vi "Dashboard Loop.vi"() -> ()   [LabVIEW 2013]
uses:
  Common Code/Dashboard UDP/Indicator Packet.ctl
  Common Code/Dashboard UDP/Auton Indicators.ctl
  Common Code/Dashboard UDP/Roller Indicators.ctl
  Common Code/IR Logic State.ctl
  Common Code/Dashboard UDP/Shooter Indicators.ctl
  Common Code/Shooter State.ctl
  Common Code/Dashboard UDP/Halo Indicators.ctl
  Common Code/Dashboard UDP/Drive Indicators.ctl
  Sensors/Encoder Data.ctl
  Sensors/Single Encoder Data.ctl
  Common Code/Vision Mode.ctl
  Drivetrain/DT Mode.ctl
  Rollers/Roller Mode.ctl
  Robot Global Data.vi
  <vilib>/Rock Robotics/WPI/Gyro/WPI_GyroRefNum Registry Get.vi
  <vilib>/Rock Robotics/WPI/Gyro/WPI_GyroGetAngle.vi
  <vilib>/Rock Robotics/WPI/DigitalInput/WPI_DigitalInputRefNum Registry Get.vi
  <vilib>/Rock Robotics/WPI/DigitalInput/WPI_DigitalInputGetValue.vi
panel:
  out "Indicator Packet":T1={"Gyro/Steer Target"=0.0, "Gyro/In Range"=FALSE, "Gyro Heading"=0.0, "Auton/Files"="", "Auton Indicators"={"DistDrive/Steer"=FALSE, "DistDrive/Y Check"=FALSE, "Auton/Left Hot"=FALSE, "Auton/Right Hot"=FALSE, "DistDrive/Y Dist"=0.0, "DistDrive/Y Target"=0.0, "DistDrive/X Dist"=0.0, "DistDrive/X Target"=0.0, "Gyro Heading"=0.0, "DistDrive/Steer Target"=0.0, "DistDrive/X Check"=FALSE, "Auton/Hot Found"=FALSE, "Auton/Goals Used"=0.0, "Auton/Total Commands"=0.0, "Auton/Current Command"=0.0, "Auton/File"=0.0}, "Heartbeat"=0.0, "100ms Loop Time"=0, "IR Dist/Line Detected Left"=FALSE, "IR Dist/Line Detected Right"=FALSE, "Roller Indicators"={"Roller/Front IR"=FALSE, "Roller/Center IR"=FALSE, "Roller/Back IR"=FALSE, "Roller/IR State"=enum."Waiting", "Roller/Auto Enabled"=FALSE, "Roller/Hold"=FALSE, "Roller/Net Solenoid"=FALSE}, "Shooter/Indicators"={"Pressure/Line"=-1.0, "Pressure/Shooter"=-1.0, "Shooter/Release"=FALSE, "Shooter/Trigger"=FALSE, "Shooter/Retracted"=FALSE, "Shooter/Ready"=FALSE, "Shooter/Add"=FALSE, "Shooter/State"=enum."Wait", "Shooter/Punch"=FALSE, "Shooter/High"=FALSE, "Shooter/AutoPunch"=FALSE}, "Halo/Indicators"={"Halo"=FALSE, "Roller Halo"=FALSE, "Shooter Halo"=FALSE, "Auto Halo"=FALSE, "Manual Halo"=FALSE}, "Drive Indicators"={"Drive/Throttle"=0.0, "Drive/Steer"=0.0, "Drive/Translation X"=0.0, "Drive/Omni"=FALSE, "Roller/Front Output"=0.0, "Roller/Back Output"=0.0, "Roller/Front Solenoid"=FALSE, "Roller/Back Solenoid"=FALSE, "Drive/Gear"=0.0}, "Encoder Data"={"Avg Distance L/R"=0.0, "Avg Speed L/R"=0.0, "Left"={"Distance"=0.0, "Speed"=0.0, "Ticks"=0.0}, "Right"={"Distance"=0.0, "Speed"=0.0, "Ticks"=0.0}, "Omni"={"Distance"=0.0, "Speed"=0.0, "Ticks"=0.0}}, "Vision Mode "=enum."Normal", "Drivetrain Mode"=enum."Manual"} {"Encoder Data"."Omni"."Ticks" format="%#.6g"; "Encoder Data"."Right"."Ticks" format="%#.6g"; "Encoder Data"."Left"."Ticks" format="%#.6g"; "Drive Indicators"."Roller/Back Output" scale=-1.0..1.0; "Drive Indicators"."Roller/Front Output" scale=-1.0..1.0; "Drive Indicators"."Drive/Translation X" scale=-1.0..1.0; "Drive Indicators"."Drive/Steer" scale=-1.0..1.0; "Drive Indicators"."Drive/Throttle" scale=-1.0..1.0}
  # "IR"
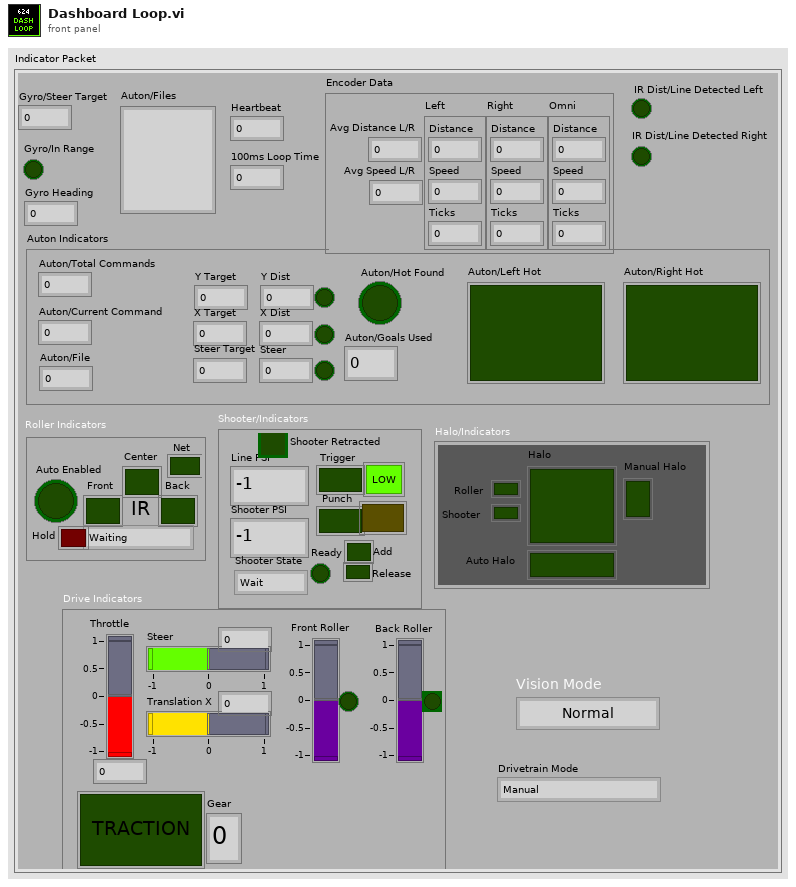
[diagram p1: front panel]
types:
  T1 = typedef "Indicator Packet.ctl" = cluster{"Gyro/Steer Target":dbl, "Gyro/In Range":bool, "Gyro Heading":dbl, "Auton/Files":string, "Auton Indicators":T2, "Heartbeat":dbl, "100ms Loop Time":i32, "IR Dist/Line Detected Left":bool, "IR Dist/Line Detected Right":bool, "Roller Indicators":T3, "Shooter/Indicators":T5, "Halo/Indicators":T7, "Drive Indicators":T8, "Encoder Data":T9, "Vision Mode ":T11, "Drivetrain Mode":T12}
  T2 = typedef "Auton Indicators.ctl" = cluster{"DistDrive/Steer":bool, "DistDrive/Y Check":bool, "Auton/Left Hot":bool, "Auton/Right Hot":bool, "DistDrive/Y Dist":dbl, "DistDrive/Y Target":dbl, "DistDrive/X Dist":dbl, "DistDrive/X Target":dbl, "Gyro Heading":dbl, "DistDrive/Steer Target":dbl, "DistDrive/X Check":bool, "Auton/Hot Found":bool, "Auton/Goals Used":dbl, "Auton/Total Commands":dbl, "Auton/Current Command":dbl, "Auton/File":dbl}
  T3 = typedef "Roller Indicators.ctl" = cluster{"Roller/Front IR":bool, "Roller/Center IR":bool, "Roller/Back IR":bool, "Roller/IR State":T4, "Roller/Auto Enabled":bool, "Roller/Hold":bool, "Roller/Net Solenoid":bool}
  T4 = typedef "IR Logic State.ctl" = enum16{"Waiting", "Requested", "Loading", "Full", "Wait for Center", "Carry", "Full Carry", "Holding"}
  T5 = typedef "Shooter Indicators.ctl" = cluster{"Pressure/Line":dbl, "Pressure/Shooter":dbl, "Shooter/Release":bool, "Shooter/Trigger":bool, "Shooter/Retracted":bool, "Shooter/Ready":bool, "Shooter/Add":bool, "Shooter/State":T6, "Shooter/Punch":bool, "Shooter/High":bool, "Shooter/AutoPunch":bool}
  T6 = typedef "Shooter State.ctl" = enum16{"Wait", "Fill Piston", "Lift Halo", "Trigger", "Reset", "Soft Release", "Soft Unpin", "Soft Refill", "Soft Shoot", "Toss Prep", "Toss Release"}
  T7 = typedef "Halo Indicators.ctl" = cluster{"Halo":bool, "Roller Halo":bool, "Shooter Halo":bool, "Auto Halo":bool, "Manual Halo":bool}
  T8 = typedef "Drive Indicators.ctl" = cluster{"Drive/Throttle":dbl, "Drive/Steer":dbl, "Drive/Translation X":dbl, "Drive/Omni":bool, "Roller/Front Output":dbl, "Roller/Back Output":dbl, "Roller/Front Solenoid":bool, "Roller/Back Solenoid":bool, "Drive/Gear":dbl}
  T9 = typedef "Encoder Data.ctl" = cluster{"Avg Distance L/R":dbl, "Avg Speed L/R":dbl, "Left":T10, "Right":T10, "Omni":T10}
  T10 = typedef "Single Encoder Data.ctl" = cluster{"Distance":dbl, "Speed":dbl, "Ticks":dbl}
  T11 = typedef "Vision Mode.ctl" = enum16{"Normal", "Extreme Left", "Extreme Right"}
  T12 = typedef "DT Mode.ctl" = enum16{"Manual", "Gyro Steer", "Distance Drive", "Fieldcentric", "Roll Maneuver", "Alt Roll Maneuver"}
  T13 = typedef "Roller Mode.ctl" = enum16{"None", "Front", "Back", "Both", "Manual"}
  T14 = typedef "WPI_DriverStationRobotMode2.ctl" = enum16{"Autonomous Disabled", "Autonomous Enabled", "Teleop Disabled", "Teleop Enabled", "Timeout", "Finish", "Test Disabled", "Test Enabled"}
  T15 = typedef "Roller Control.ctl" = cluster{"Mode":T13, "Front":enum16{"Stop", "Forward", "Reverse"}, "Back":enum16{"Stop", "Forward", "Reverse"}, "Reset":bool, "Front Piston":bool, "Halo":bool, "Net Piston":bool, "Carry Two":bool, "Hold":bool}
  T16 = typedef "Drivetrain Status.ctl" = cluster{"Mode":T12, "X":dbl, "Y":dbl, "Steer":dbl, "Low Gear":bool, "Omni":bool}
  T17 = typedef "Roller Status.ctl" = cluster{"State":T4, "Front Power":dbl, "Front Solenoid":bool}
  T18 = typedef "Distance Drive Result.ctl" = cluster{"Finished":bool, "distance target":cluster{"x":dbl, "y":dbl}, "Heading Target":dbl, "X Check":bool, "Y Check":bool, "X Dist":dbl, "Y Dist":dbl}
  T19 = typedef "Shooter Manual Control.ctl" = cluster{"Command":T20, "Offset":dbl, "Trigger":bool, "Add":bool, "Release":bool, "Reset":bool, "Target Pressure":dbl, "Punch":bool, "AutoPunch":bool}
  T20 = typedef "Shooter Command.ctl" = enum16{"None", "Warmup", "Shoot", "Line Shoot", "Soft Shoot", "Toss"}
  T21 = typedef "Dashboard UDP Packet.ctl" = cluster{"Camera":T22, "Gyro":T23, "Encoder":T25, "Auto Shift":T26, "Auton":T27, "Drive/Ramp X":dbl, "Drive/Ramp Y":dbl, "Drive/Battery Cutoff":dbl, "Pressure/Compressor Min Voltage":dbl, "Pressure/Compressor Delay":dbl, "Controller/Strafe Correction":bool, "Shooter":T28, "Rollers":T29, "Abort":bool, "Finish":bool, "IR Halo Sustain Time":dbl, "Disable Compressor":bool, "Center Omni Drive Delay":i32, "Vision Mode":T11, "Radius Throttle":bool, "Fieldcentric":T30, "Roll":T31, "Stick Deadband":dbl}
  T22 = typedef "Camera Controls.ctl" = cluster{"Camera/View Angle X":dbl, "Camera/Goal Track Timeout":dbl, "Camera/View Angle Y":dbl, "Camera/Goal Exposure":dbl, "Camera/Vision Receive Timeout":dbl, "Camera/Offset 1":dbl, "Camera/Offset 2":dbl}
  T23 = typedef "Gyro Controls.ctl" = cluster{"Gyro/Angle Tolerance":dbl, "Gyro/Steer Closeness Threshold":dbl, "Steer PID":T24, "Steer Close PID":T24}
  T24 = typedef "PID Params.ctl" = cluster{"max":dbl, "min":dbl, "P":dbl, "I":dbl, "D":dbl}
  T25 = typedef "Encoder Controls.ctl" = cluster{"Encoders/Reset":bool, "Encoders/Omni Constant":dbl, "Encoders/Omni Tick Constant":dbl, "Encoders/Left Constant":dbl, "Encoders/Right Constant":dbl, "Encoders/Right Tick Constant":dbl}
  T26 = typedef "Auto Shift Controls.ctl" = cluster{"AutoShift/Upshift Throttle Accel":dbl, "AutoShift/Speed Threshold":dbl, "AutoShift/Upshift Throttle":dbl, "AutoShift/Upshift Accel":dbl, "AutoShift/Downshift Accel":dbl, "AutoShift/Downshift Throttle":dbl, "AutoShift/Delay":dbl, "AutoShift/Enabled":bool}
  T27 = typedef "Auton Controls.ctl" = cluster{"Auton/Left Shoot X-Coord":dbl, "Auton/Right Shoot X-Coord":dbl, "DistDrive/Distance Stop Threshold":dbl, "DistDrive/Max Stop Speed":dbl, "Auton/Back Piston Time":dbl, "Auton/Manual Hot":bool, "Auton/Manual Hot Right":bool, "Default X PID":T24, "Default Y PID":T24, "Half Over Delay":dbl}
  T28 = typedef "Shooter Controls.ctl" = cluster{"Shooter/Reset Time":dbl, "Shooter/Release Delay":dbl, "Shooter/Pressure Steady Time":dbl, "Shooter/Misfire Delay":dbl, "Shooter/Ball Settle Time":dbl, "Shooter/Line IR Delay":dbl, "Pressure/Upper PSI Time":dbl, "Pressure/Lower PSI Time":dbl, "Shooter/Punch Delay":dbl, "Shooter/Target Pressure":dbl, "Pressure/Line B":dbl, "Pressure/Line M":dbl, "Pressure/Shooter M":dbl, "Pressure/Shooter B":dbl, "Halo Time":dbl, "Soft Release Delay":dbl, "Soft Unpin Delay":dbl, "Soft Shoot Delay":dbl, "Toss Release Time":dbl}
  T29 = typedef "Roller Controls.ctl" = cluster{"Roller/Load IRs Verify Time":dbl, "Roller/Center IR Latch Time":dbl, "Roller/Speed Front":dbl, "Roller/Speed Back":dbl, "Roller/Entry Timeout":dbl, "Roller/To Center Timeout":dbl, "Roller/Sustain Time":dbl, "Roller/Verify Center Time":dbl}
  T30 = typedef "Fieldcentric Controls.ctl" = cluster{"Relative Angle":bool, "Point Robot":bool, "X/Y ratio low":dbl, "Steering Gain":dbl, "Force Omni Down":bool, "Enable":bool, "X/Y ratio high":dbl}
  T31 = typedef "Roll Maneuver.ctl" = cluster{"X 1":dbl, "Y 1":dbl, "Y 2":dbl, "X 2":dbl, "Y 3":dbl, "X 3":dbl, "Time 1":i32, "Time 2":i32, "Time 3":i32, "Angle Start":dbl, "Angle End":dbl, "Angle Linearity":dbl}
  T32 = typedef "Shooter Status.ctl" = cluster{"Shooter Ready":bool, "Add":bool, "Punch":bool, "Release":bool, "Trigger":bool, "High":bool, "State":T6}
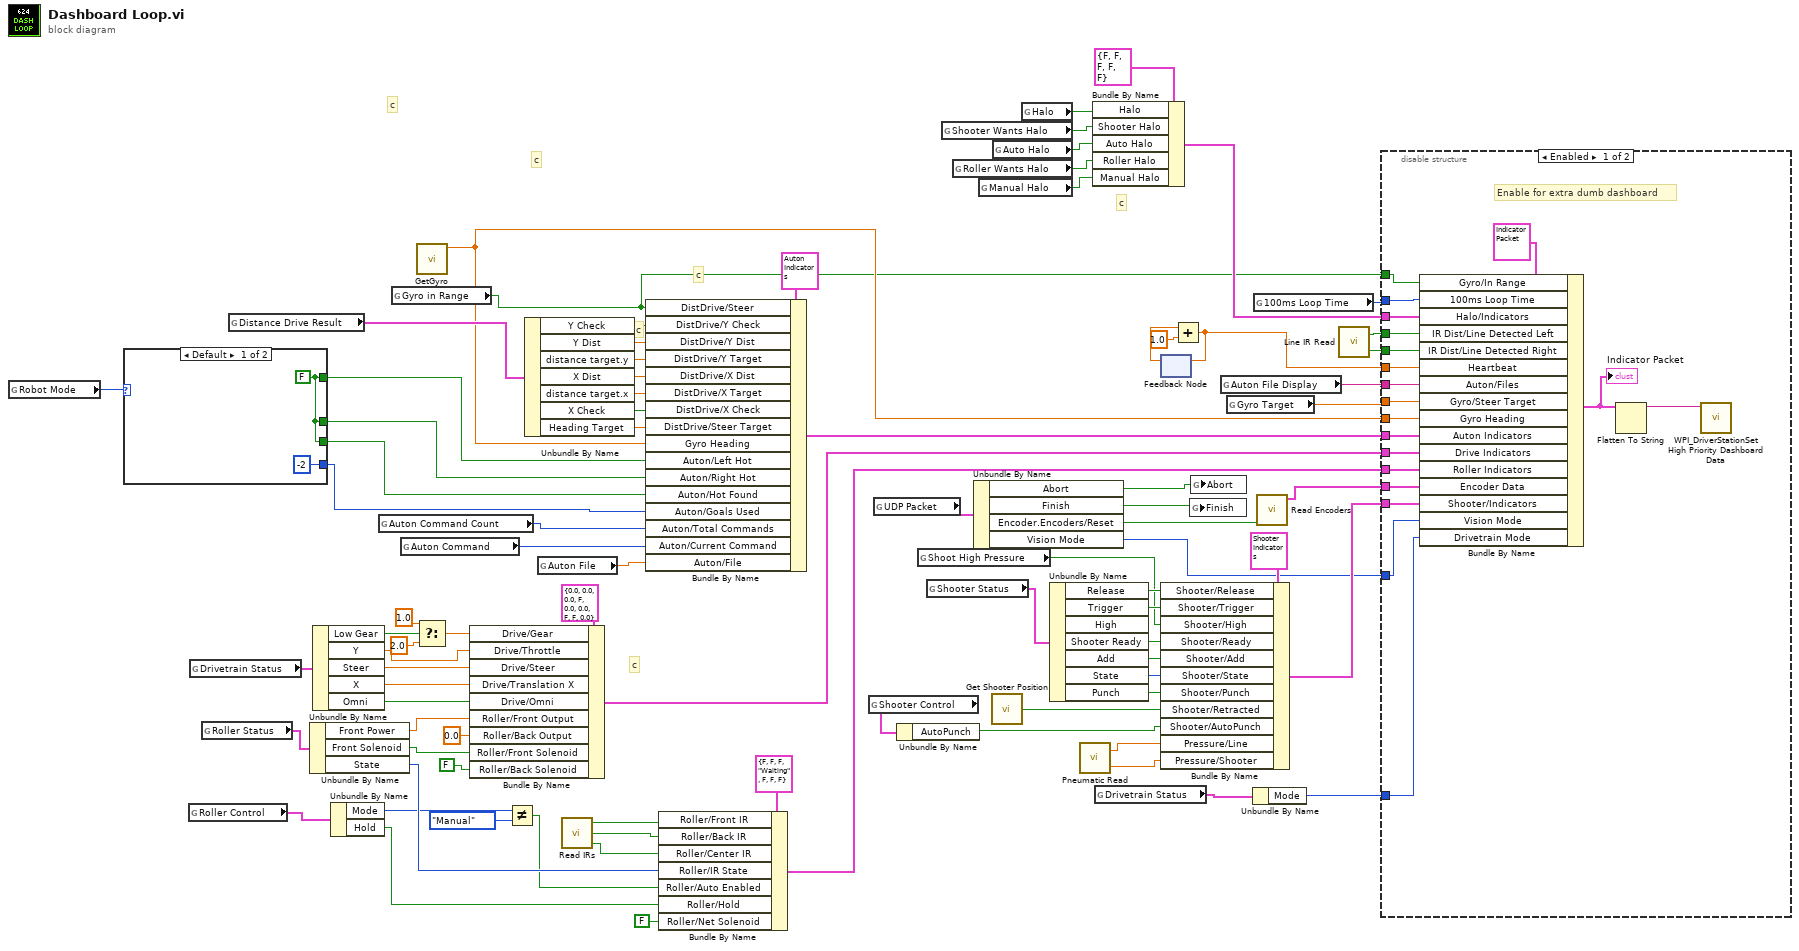
[diagram p0: block diagram]
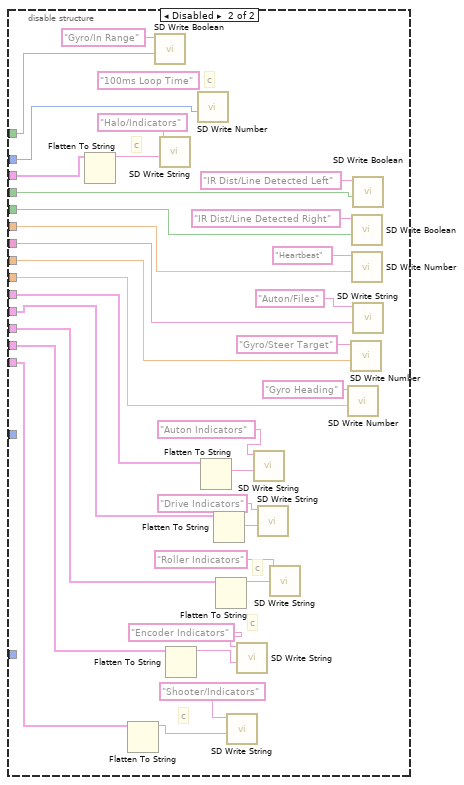
[diagram p2: hidden frame]
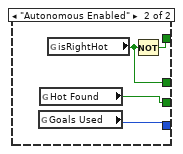
[diagram p3: hidden frame]
diagram:
  # "c"
  # "c"
  # "c"
  # "c"
  # "c"
  # "c"
  n1 = global read "Robot Global Data.vi" "Robot Mode"() -> (w82:T14)
  n2 = case shown="Default" w82 {
    tunnel: [w88 w92] -> w33
    tunnel: [w88 w91] -> w34
    tunnel: [w88 w90] -> w35
    tunnel: [-2 ("Goals Used") w89] -> w36
    frame Default {
      w88 = FALSE
    }
    frame "Autonomous Enabled" {
      n3 = global read "Robot Global Data.vi" "Goals Used"() -> (w89:i32)
      n4 = global read "Robot Global Data.vi" "Hot Found"() -> (w90:bool)
      n5 = global read "Robot Global Data.vi" "isRightHot"() -> (w91:bool)
      n6 = Not(x=w91) -> (.not. x?=w92:bool)
    }
  }
  n7 = global read "Robot Global Data.vi" "Roller Control"() -> (w57:T15)
  n8 = global read "Robot Global Data.vi" "Drivetrain Status"() -> (w76:T16)
  n9 = global read "Robot Global Data.vi" "Roller Status"() -> (w69:T17)
  n10 = global read "Robot Global Data.vi" "Distance Drive Result"() -> (w32:T18)
  n11 = Unbundle By Name(w69) -> ("Front Power"=w67:dbl, "Front Solenoid"=w68:bool, "State"=w61:T4)
  n12 = Unbundle By Name(w76) -> ("Low Gear"=w75:bool, "Y"=w73:dbl, "Steer"=w72:dbl, "X"=w71:dbl, "Omni"=w70:bool)
  n13 = Unbundle By Name(w57) -> ("Mode"=w56:T13, "Hold"=w53:bool)
  n14 = global read "Robot Global Data.vi" "Auton Command Count"() -> (w37:i32)
  n15 = global read "Robot Global Data.vi" "Gyro in Range"() -> (w5:bool)
  n16 = global read "Robot Global Data.vi" "Auton Command"() -> (w38:i32)
  n17 = call "GetGyro.vi"() -> ("Angle"=w13:dbl)  [unwired: 9 in, 2 out]
  n18 = Select(t=1.0, s=w75, f=2.0) -> (s? t:f=w74:dbl)
  n19 = Bundle By Name(cluster=T8 {"Drive/Throttle"=0.0, "Drive/Steer"=0.0, "Drive/Translation X"=0.0, "Drive/Omni"=FALSE, "Roller/Front Output"=0.0, "Roller/Back Output"=0.0, "Roller/Front Solenoid"=FALSE, "Roller/Back Solenoid"=FALSE, "Drive/Gear"=0.0} ("Drive Indicators"), "Drive/Gear"=w74, "Drive/Throttle"=w73, "Drive/Steer"=w72, "Drive/Translation X"=w71, "Drive/Omni"=w70, "Roller/Front Output"=w67, "Roller/Back Output"=0.0, "Roller/Front Solenoid"=w68, "Roller/Back Solenoid"=FALSE) -> (w11:T8)
  n20 = Not Equal?(x=w56, y=Roller_Mode."Manual") -> (x != y?=w54:bool)
  n21 = Unbundle By Name(w32) -> ("Y Check"=w25:bool, "Y Dist"=w26:dbl, "distance target.y"=w27:dbl, "X Dist"=w28:dbl, "distance target.x"=w29:dbl, "X Check"=w30:bool, "Heading Target"=w31:dbl)
  n22 = global read "Robot Global Data.vi" "Auton File"() -> (w39:dbl)
  n23 = call "Read IRs.vi"() -> ("Center"=w58:bool, "Back"=w59:bool, "Front"=w60:bool)  [unwired: 2 in, 1 out]
  n24 = Bundle By Name(cluster=T2 {"DistDrive/Steer"=FALSE, "DistDrive/Y Check"=FALSE, "Auton/Left Hot"=FALSE, "Auton/Right Hot"=FALSE, "DistDrive/Y Dist"=0.0, "DistDrive/Y Target"=0.0, "DistDrive/X Dist"=0.0, "DistDrive/X Target"=0.0, "Gyro Heading"=0.0, "DistDrive/Steer Target"=0.0, "DistDrive/X Check"=FALSE, "Auton/Hot Found"=FALSE, "Auton/Goals Used"=0.0, "Auton/Total Commands"=0.0, "Auton/Current Command"=0.0, "Auton/File"=0.0} ("Auton Indicators"), "DistDrive/Steer"=w5, "DistDrive/Y Check"=w25, "DistDrive/Y Dist"=w26, "DistDrive/Y Target"=w27, "DistDrive/X Dist"=w28, "DistDrive/X Target"=w29, "DistDrive/X Check"=w30, "DistDrive/Steer Target"=w31, "Gyro Heading"=w13, "Auton/Left Hot"=w33, "Auton/Right Hot"=w34, "Auton/Hot Found"=w35, "Auton/Goals Used"=w36, "Auton/Total Commands"=w37, "Auton/Current Command"=w38, "Auton/File"=w39) -> (w12:T2)
  n25 = Bundle By Name(cluster=T3 {"Roller/Front IR"=FALSE, "Roller/Center IR"=FALSE, "Roller/Back IR"=FALSE, "Roller/IR State"=enum."Waiting", "Roller/Auto Enabled"=FALSE, "Roller/Hold"=FALSE, "Roller/Net Solenoid"=FALSE} ("Roller Indicators"), "Roller/Front IR"=w60, "Roller/Back IR"=w59, "Roller/Center IR"=w58, "Roller/IR State"=w61, "Roller/Auto Enabled"=w54, "Roller/Hold"=w53, "Roller/Net Solenoid"=FALSE) -> (w10:T3)
  n26 = global read "Robot Global Data.vi" "Shooter Control"() -> (w81:T19)
  n27 = global read "Robot Global Data.vi" "UDP Packet"() -> (w80:T21)
  n28 = Unbundle By Name(w81) -> ("AutoPunch"=w43:bool)
  n29 = global read "Robot Global Data.vi" "Shoot High Pressure"() -> (w24:bool)
  n30 = global read "Robot Global Data.vi" "Shooter Status"() -> (w51:T32)
  n31 = global read "Robot Global Data.vi" "Shooter Wants Halo"() -> (w19:bool)
  n32 = global read "Robot Global Data.vi" "Roller Wants Halo"() -> (w21:bool)
  n33 = Unbundle By Name(w80) -> ("Abort"=w79:bool, "Finish"=w78:bool, "Encoder.Encoders/Reset"=w77:bool, "Vision Mode"=w3:T11)
  n34 = global read "Robot Global Data.vi" "Manual Halo"() -> (w22:bool)
  n35 = call "Get Shooter Position.vi"() -> ("Is Retracted"=w44:bool)  [unwired: 1 in]
  n36 = global read "Robot Global Data.vi" "Auto Halo"() -> (w20:bool)
  n37 = global read "Robot Global Data.vi" "Halo"() -> (w18:bool)
  n38 = Unbundle By Name(w51) -> ("Release"=w50:bool, "Trigger"=w49:bool, "Shooter Ready"=w48:bool, "Add"=w47:bool, "State"=w46:T6, "Punch"=w45:bool)  [unwired: 1 out]
  n39 = call "Pneumatic Read.vi"() -> ("Shooter"=w41:dbl, "Line"=w42:dbl)  [unwired: 2 in]
  n40 = Bundle By Name(cluster=T7 {"Halo"=FALSE, "Roller Halo"=FALSE, "Shooter Halo"=FALSE, "Auto Halo"=FALSE, "Manual Halo"=FALSE} ("Halo Indicators"), "Halo"=w18, "Shooter Halo"=w19, "Auto Halo"=w20, "Roller Halo"=w21, "Manual Halo"=w22) -> (w16:T7)
  n41 = global read "Robot Global Data.vi" "Drivetrain Status"() -> (w2:T16)
  n42 = feedback #1() -> (w85:dbl)  [unwired: 1 in]
  n43 = Bundle By Name(cluster=T5 {"Pressure/Line"=-1.0, "Pressure/Shooter"=-1.0, "Shooter/Release"=FALSE, "Shooter/Trigger"=FALSE, "Shooter/Retracted"=FALSE, "Shooter/Ready"=FALSE, "Shooter/Add"=FALSE, "Shooter/State"=enum."Wait", "Shooter/Punch"=FALSE, "Shooter/High"=FALSE, "Shooter/AutoPunch"=FALSE} ("Shooter Indicators"), "Shooter/Release"=w50, "Shooter/Trigger"=w49, "Shooter/High"=w24, "Shooter/Ready"=w48, "Shooter/Add"=w47, "Shooter/State"=w46, "Shooter/Punch"=w45, "Shooter/Retracted"=w44, "Shooter/AutoPunch"=w43, "Pressure/Line"=w42, "Pressure/Shooter"=w41) -> (w9:T5)
  n44 = Add(x=w85, y=1.0) -> (x+y=w15:dbl)
  n45 = feedback-in #1(w15) -> ()
  n46 = global write "Robot Global Data.vi" "Finish"(w78) -> ()
  n47 = global write "Robot Global Data.vi" "Abort"(w79) -> ()
  n48 = global read "Robot Global Data.vi" "Auton File Display"() -> (w6:string)
  n49 = global read "Robot Global Data.vi" "Gyro Target"() -> (w14:dbl)
  n50 = Unbundle By Name(w2) -> ("Mode"=w1:T12)
  n51 = global read "Robot Global Data.vi" "100ms Loop Time"() -> (w17:i32)
  n52 = call "Read Encoders.vi"("Reset"=w77) -> ("Encoder Data"=w4:T9)  [unwired: 10 in]
  n53 = call "Line IR Read.vi"() -> ("Line IR Right"=w7:bool, "Line IR Left"=w8:bool)  [unwired: 2 in]
  n54 = disable-structure shown="Enabled" {
    disable-tunnel: w17 -> [w110 w144]
    disable-tunnel: w16 -> [w109 w141]
    disable-tunnel: w8 -> [w108 w139]
    disable-tunnel: w7 -> [w107 w138]
    disable-tunnel: w15 -> [w106 w135]
    disable-tunnel: w6 -> [w105 w133]
    disable-tunnel: w14 -> [w104 w131]
    disable-tunnel: w13 -> [w103 w129]
    disable-tunnel: w12 -> [w102 w126]
    disable-tunnel: w11 -> [w101 w120]
    disable-tunnel: w10 -> [w100 w123]
    disable-tunnel: w4 -> [w95 w117]
    disable-tunnel: w9 -> [w99 w114]
    disable-tunnel: w5 -> [w96 w112]
    disable-tunnel: w3 -> [w94 _]
    disable-tunnel: w1 -> [w93 _]
    frame Enabled {
      # "Enable for extra dumb dashboard"
      n55 = Bundle By Name(cluster=T1 {"Gyro/Steer Target"=0.0, "Gyro/In Range"=FALSE, "Gyro Heading"=0.0, "Auton/Files"="", "Auton Indicators"={"DistDrive/Steer"=FALSE, "DistDrive/Y Check"=FALSE, "Auton/Left Hot"=FALSE, "Auton/Right Hot"=FALSE, "DistDrive/Y Dist"=0.0, "DistDrive/Y Target"=0.0, "DistDrive/X Dist"=0.0, "DistDrive/X Target"=0.0, "Gyro Heading"=0.0, "DistDrive/Steer Target"=0.0, "DistDrive/X Check"=FALSE, "Auton/Hot Found"=FALSE, "Auton/Goals Used"=0.0, "Auton/Total Commands"=0.0, "Auton/Current Command"=0.0, "Auton/File"=0.0}, "Heartbeat"=0.0, "100ms Loop Time"=0, "IR Dist/Line Detected Left"=FALSE, "IR Dist/Line Detected Right"=FALSE, "Roller Indicators"={"Roller/Front IR"=FALSE, "Roller/Center IR"=FALSE, "Roller/Back IR"=FALSE, "Roller/IR State"=enum."Waiting", "Roller/Auto Enabled"=FALSE, "Roller/Hold"=FALSE, "Roller/Net Solenoid"=FALSE}, "Shooter/Indicators"={"Pressure/Line"=0.0, "Pressure/Shooter"=0.0, "Shooter/Release"=FALSE, "Shooter/Trigger"=FALSE, "Shooter/Retracted"=FALSE, "Shooter/Ready"=FALSE, "Shooter/Add"=FALSE, "Shooter/State"=enum."Wait", "Shooter/Punch"=FALSE, "Shooter/High"=FALSE, "Shooter/AutoPunch"=FALSE}, "Halo/Indicators"={"Halo"=FALSE, "Roller Halo"=FALSE, "Shooter Halo"=FALSE, "Auto Halo"=FALSE, "Manual Halo"=FALSE}, "Drive Indicators"={"Drive/Throttle"=0.0, "Drive/Steer"=0.0, "Drive/Translation X"=0.0, "Drive/Omni"=FALSE, "Roller/Front Output"=0.0, "Roller/Back Output"=0.0, "Roller/Front Solenoid"=FALSE, "Roller/Back Solenoid"=FALSE, "Drive/Gear"=0.0}, "Encoder Data"={"Avg Distance L/R"=0.0, "Avg Speed L/R"=0.0, "Left"={"Distance"=0.0, "Speed"=0.0, "Ticks"=0.0}, "Right"={"Distance"=0.0, "Speed"=0.0, "Ticks"=0.0}, "Omni"={"Distance"=0.0, "Speed"=0.0, "Ticks"=0.0}}, "Vision Mode "=enum."Normal", "Drivetrain Mode"=enum."Manual"} ("Indicator Packet"), "Gyro/In Range"=w96, "100ms Loop Time"=w110, "Halo/Indicators"=w109, "IR Dist/Line Detected Left"=w108, "IR Dist/Line Detected Right"=w107, "Heartbeat"=w106, "Auton/Files"=w105, "Gyro/Steer Target"=w104, "Gyro Heading"=w103, "Auton Indicators"=w102, "Drive Indicators"=w101, "Roller Indicators"=w100, "Encoder Data"=w95, "Shooter/Indicators"=w99, "Vision Mode"=w94, "Drivetrain Mode"=w93) -> (w98:T1)
      "Indicator Packet" <- w98
      n56 = Flatten To String(anything=w98) -> (data string=w97:string)  [unwired: 3 in, 2 out]
      n57 = call <vilib>:"WPI_DriverStationSet High Priority Dashboard Data.vi"("User Data"=w97) -> ()  [unwired: 10 in, 1 out]
    }
    frame Disabled {
      (unwired) "100ms Loop Time" ("Name")
      # "c"
      # "c"
      # "c"
      # "c"
      # "c"
      n58 = Flatten To String(anything=w141) -> (data string=w142:string)  [unwired: 3 in, 2 out]
      n59 = Flatten To String(anything=w114) -> (data string=w115:string)  [unwired: 3 in, 2 out]
      n60 = call <vilib>:"SD Write Boolean.vi"("Boolean"=w112, "Name"="Gyro/In Range") -> ()  [unwired: 8 in, 2 out]
      n61 = call <vilib>:"SD Write String.vi"("String"=w142, "Name"="Halo/Indicators") -> ()  [unwired: 8 in, 2 out]
      n62 = Flatten To String(anything=w117) -> (data string=w118:string)  [unwired: 3 in, 2 out]
      n63 = call <vilib>:"SD Write Number.vi"("Numeric"=w144) -> ()  [unwired: 9 in, 2 out]
      n64 = Flatten To String(anything=w126) -> (data string=w128:string)  [unwired: 3 in, 2 out]
      n65 = Flatten To String(anything=w120) -> (data string=w121:string)  [unwired: 3 in, 2 out]
      n66 = Flatten To String(anything=w123) -> (data string=w124:string)  [unwired: 3 in, 2 out]
      n67 = call <vilib>:"SD Write String.vi"("String"=w115, "Name"="Shooter/Indicators") -> ()  [unwired: 8 in, 2 out]
      n68 = call <vilib>:"SD Write String.vi"("String"=w118, "Name"="Encoder Indicators") -> ()  [unwired: 8 in, 2 out]
      n69 = call <vilib>:"SD Write String.vi"("String"=w128, "Name"="Auton Indicators") -> ()  [unwired: 8 in, 2 out]
      n70 = call <vilib>:"SD Write String.vi"("String"=w121, "Name"="Drive Indicators") -> ()  [unwired: 8 in, 2 out]
      n71 = call <vilib>:"SD Write String.vi"("String"=w124, "Name"="Roller Indicators") -> ()  [unwired: 8 in, 2 out]
      n72 = call <vilib>:"SD Write Number.vi"("Numeric"=w129, "Name"="Gyro Heading") -> ()  [unwired: 8 in, 2 out]
      n73 = call <vilib>:"SD Write Number.vi"("Numeric"=w131, "Name"="Gyro/Steer Target") -> ()  [unwired: 8 in, 2 out]
      n74 = call <vilib>:"SD Write Boolean.vi"("Boolean"=w138, "Name"="IR Dist/Line Detected Right") -> ()  [unwired: 8 in, 2 out]
      n75 = call <vilib>:"SD Write Number.vi"("Numeric"=w135, "Name"="Heartbeat") -> ()  [unwired: 8 in, 2 out]
      n76 = call <vilib>:"SD Write Boolean.vi"("Boolean"=w139, "Name"="IR Dist/Line Detected Left") -> ()  [unwired: 8 in, 2 out]
      n77 = call <vilib>:"SD Write String.vi"("String"=w133, "Name"="Auton/Files") -> ()  [unwired: 8 in, 2 out]
    }
  }
